vi "beginPreparePassPlay.vi"(8 "error in (no error)":errorcluster, 9 "last command_interpreted":T1, 10 "Game":refnum<class "Game.lvclass">, 11 "PreparePassPlay in":refnum<class "PreparePassPlay.lvclass">) -> (0 "error out":errorcluster, 2 "Boolean":bool, 3 "PreparePassPlay out":refnum<class "PreparePassPlay.lvclass">)   [LabVIEW 2018, in "PreparePassPlay.lvclass"]
uses:
  PreparePassPlay.lvclass
  Game_class/Game.lvclass
  Referee_class/command_interpreted.ctl
  Game_class/Game.lvclass/Game.ctl
  Referee_class/Referee.lvclass/Referee.ctl
  Game_class/Read Referee.vi
  Referee_class/Read command_interpreted.vi
  Referee_class/Referee.lvclass
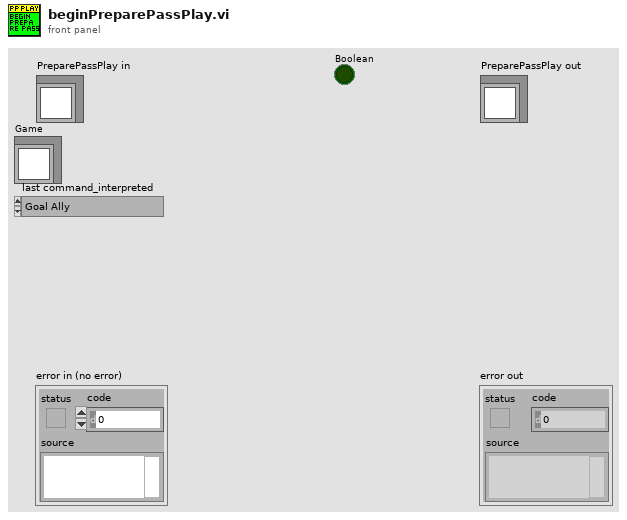
[diagram p1: front panel]
types:
  T1 = typedef "command_interpreted.ctl" = enum16{"Goal Ally", "Goal Enemy", "Ball Placement Enemy", "Ball Placement Ally", "Normal Half Time", "Extra Time  Break", "Extra Half Time", "None", "Post Game", "PKA Normal Start", "Prepare Kickoff Ally", "PKE Normal Start", "Prepare Kickoff Enemy", "Force Start", "Halt", "Timeout", "Prepare Penalty Ally", "Prepare Penalty Enemy", "PPA NormalStart", "PPE Normal Start", "Indirect Free Ally", "Direct Free Enemy", "Direct Free Ally", "Indirect Free Enemy", "Stop"}
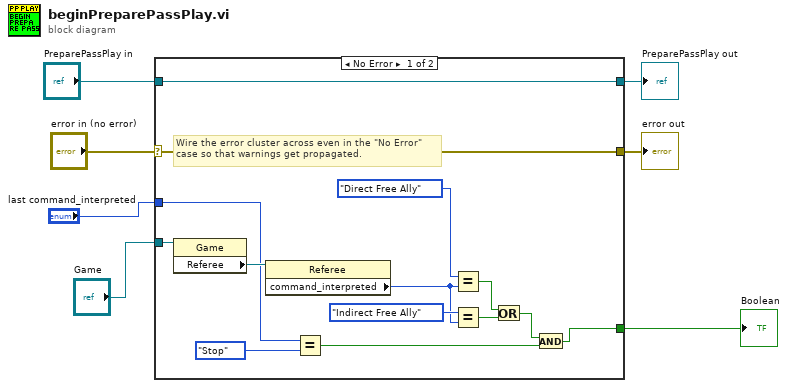
[diagram p0: block diagram]
diagram:
  n1 = case shown="No Error" "error in (no error)" {
    selector: "error in (no error)" -> [w20 w23]
    tunnel: [w20 w23] -> w6
    tunnel: [w21 w22] -> w4
    tunnel: "PreparePassPlay in" -> [w21 w22]
    tunnel: "Game" -> [w19 _]
    tunnel: [w10 _] -> w2
    tunnel: "last command_interpreted" -> [w8 _]
    frame No Error {
      # "Wire the error cluster across even in the \"No Error\"\ncase so that warnings get propagated."
      n2 = property class="Game"(reference=w19) -> ("Referee"=w18:refnum<class "Referee.lvclass">)  [unwired: 1 in, 2 out]
      n3 = property class="Referee"(reference=w18) -> ("command_interpreted"=w14:T1)  [unwired: 1 in, 2 out]
      n4 = Equal?(x=w8, y=command_interpreted."Stop" ("command_interpreted")) -> (x = y?=w9:bool)
      n5 = Equal?(x=command_interpreted."Direct Free Ally" ("command_interpreted"), y=w14) -> (x = y?=w13:bool)
      n6 = Equal?(x=command_interpreted."Indirect Free Ally" ("command_interpreted"), y=w14) -> (x = y?=w11:bool)
      n7 = Or(x=w13, y=w11) -> (x .or. y?=w12:bool)
      n8 = And(x=w12, y=w9) -> (x .and. y?=w10:bool)
    }
    frame Error {
    }
  }
  "error out" <- w6
  "PreparePassPlay out" <- w4
  "Boolean" <- w2
